vi "crh_xcopyYesterday.vi"(11 "folder":string="QAMT02\\CRH3605_95TH248") -> (0 "OK 2":bool, 1 "OK":bool, 3 "OK 3":bool)   [LabVIEW 2012]
panel:
  out "concatenated string":string
  out "concatenated string 2":string
  out "folder 2":string
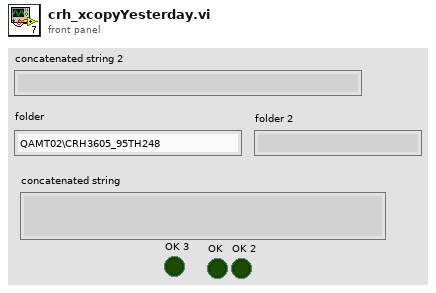
[diagram p1: front panel]
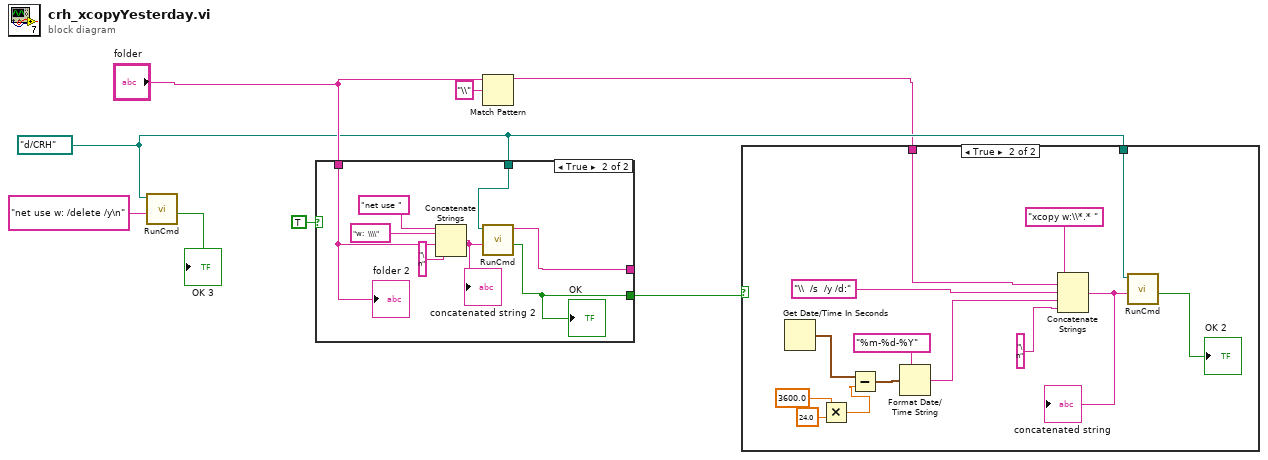
[diagram p0: block diagram]
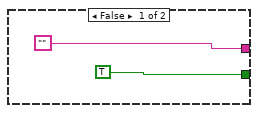
[diagram p3: hidden frame]
diagram:
  w4 = path "d:/CRH" ("working directory")
  n1 = call "RunCmd.vi"("Cmd String"="net use w: /delete /y\n" ("string"), "working directory"=w4) -> ("OK"=→"OK 3":bool)  [unwired: 8 in, 1 out]
  n2 = case shown="True" TRUE {
    tunnel: [TRUE w12] -> w6
    tunnel: ["" w13] -> _
    tunnel: "folder" -> [_ w15]
    tunnel: w4 -> [_ w14]
    frame False {
    }
    frame True {
      n3 = Concatenate Strings("net use " ("string"), "w:  \\\\" ("string"), w15, "\n" ("string")) -> (w18:string)
      "concatenated string 2" <- w18
      n4 = call "RunCmd.vi"("Cmd String"=w18, "working directory"=w14) -> ("OK"=w12:bool, "Output"=w13:string)  [unwired: 8 in]
      "OK" <- w12
      "folder 2" <- w15
    }
  }
  n5 = Match Pattern(string="folder", regular expression="\\") -> (before substring=w3:string)  [unwired: 1 in, 3 out]
  n6 = case shown="True" w6 {
    tunnel: w3 -> [_ w32]
    tunnel: w4 -> [_ w29]
    frame False {
    }
    frame True {
      n7 = Get Date/Time In Seconds() -> (seconds since 1Jan1904=w21:timestamp)
      n8 = Multiply(x=3600.0, y=24.0) -> (x*y=w23:dbl)
      n9 = Subtract(x=w21, y=w23) -> (x-y=w24:timestamp)
      n10 = Format Date/Time String(time format string (%c)="%m-%d-%Y", seconds (now)=w24) -> (date/time string=w20:string)  [unwired: 1 in]
      n11 = Concatenate Strings("xcopy w:\\*.* " ("string"), w32, "\\  /s  /y /d:" ("string"), w20, "\n" ("string")) -> (w28:string)
      "concatenated string" <- w28
      n12 = call "RunCmd.vi"("Cmd String"=w28, "working directory"=w29) -> ("OK"=→"OK 2":bool)  [unwired: 8 in, 1 out]
    }
  }
